vi "Chart-Draw Bounding.vi"(8 "error in (no error)":errorcluster, 11 "XY Graph Ref In":refnum<vi>) -> (0 "error out":errorcluster, 3 "XY Graph Ref Out":refnum<vi>)   [LabVIEW 2020]
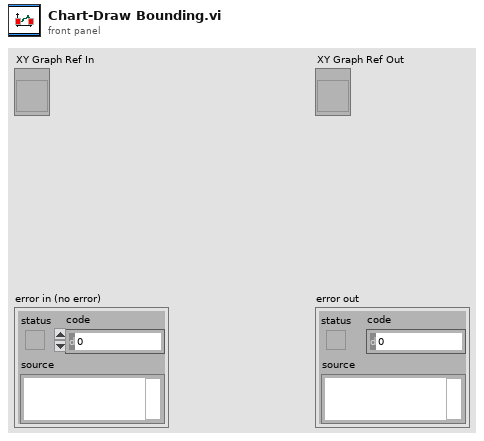
[diagram p1: front panel]
types:
  T1 = cluster{"left":i16, "top":i16, "right":i16, "bottom":i16}
  T2 = cluster{"XScale.Maximum":dbl, "XScale.Maximum":dbl}
  T3 = cluster{"XScale.Minimum":dbl, "XScale.Minimum":dbl}
  T4 = cluster{"Cursor.Cursor X":dbl, "Cursor.Cursor X":dbl}
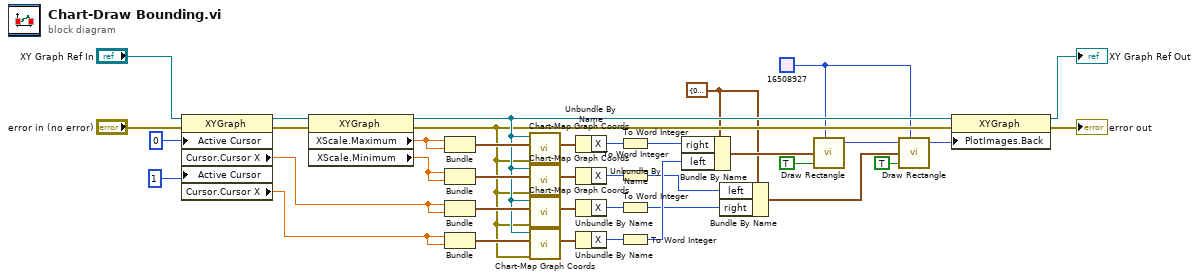
[diagram p0: block diagram]
diagram:
  w3 = u32 16508927
  w6 = T1 {"left"=0, "top"=0, "right"=0, "bottom"=500} ("rect")
  n1 = property class="XYGraph"(reference="XY Graph Ref In", error in="error in (no error)", "Active Cursor"=u32 0, "Active Cursor"=u32 1) -> (reference out=w18:refnum<vi>, error out=w19:errorcluster, "Cursor.Cursor X"=w25:dbl, "Cursor.Cursor X"=w24:dbl)
  n2 = property on="Property Node" class="XYGraph"(reference=w18, error in=w19) -> (reference out=w26:refnum<vi>, error out=w15:errorcluster, "XScale.Maximum"=w36:dbl, "XScale.Minimum"=w35:dbl)
  n3 = Bundle("XScale.Maximum"=w36, "XScale.Maximum"=w36) -> (w27:T2)  [unwired: 1 in]
  n4 = Bundle("XScale.Minimum"=w35, "XScale.Minimum"=w35) -> (w33:T3)  [unwired: 1 in]
  n5 = Bundle("Cursor.Cursor X"=w25, "Cursor.Cursor X"=w25) -> (w31:T4)  [unwired: 1 in]
  n6 = Bundle("Cursor.Cursor X"=w24, "Cursor.Cursor X"=w24) -> (w30:T4)  [unwired: 1 in]
  n7 = call "Chart-Map Graph Coords.vi"("error in (no error)"=w15, "XY"=w27, "XY Graph Ref"=w26) -> ("Coords"=w28:cluster{"X":i32, "Y":i32})  [unwired: 7 in, 1 out]
  n8 = call "Chart-Map Graph Coords.vi"("error in (no error)"=w15, "XY"=w33, "XY Graph Ref"=w26) -> ("Coords"=w34:cluster{"X":i32, "Y":i32})  [unwired: 7 in, 1 out]
  n9 = call "Chart-Map Graph Coords.vi"("error in (no error)"=w15, "XY"=w31, "XY Graph Ref"=w26) -> ("Coords"=w32:cluster{"X":i32, "Y":i32})  [unwired: 7 in, 1 out]
  n10 = call "Chart-Map Graph Coords.vi"("error in (no error)"=w15, "XY"=w30, "XY Graph Ref"=w26) -> ("Coords"=w29:cluster{"X":i32, "Y":i32})  [unwired: 7 in, 1 out]
  n11 = Unbundle By Name(w28) -> ("X"=w14:i32)
  n12 = Unbundle By Name(w34) -> ("X"=w10:i32)
  n13 = Unbundle By Name(w32) -> ("X"=w8:i32)
  n14 = Unbundle By Name(w29) -> ("X"=w12:i32)
  n15 = To Word Integer(number=w14) -> (16bit integer=w13:i16)
  n16 = To Word Integer(number=w10) -> (16bit integer=w9:i16)
  n17 = To Word Integer(number=w8) -> (16bit integer=w7:i16)
  n18 = To Word Integer(number=w12) -> (16bit integer=w11:i16)
  n19 = Bundle By Name(cluster=w6, "right"=w13, "left"=w11) -> (w23:T1)
  n20 = Bundle By Name(cluster=w6, "left"=w9, "right"=w7) -> (w5:T1)
  n21 = call <vilib>:"Draw Rectangle.vi"("rect"=w23, "fill?(F)"=TRUE, "color(black)"=w3) -> ("new picture"=w22:picture)  [unwired: 6 in]
  n22 = call <vilib>:"Draw Rectangle.vi"("picture"=w22, "rect"=w5, "fill?(F)"=TRUE, "color(black)"=w3) -> ("new picture"=w21:picture)  [unwired: 5 in]
  n23 = property on="Property Node" class="XYGraph"(reference=w26, error in=w15, "PlotImages.Back"=w21) -> (reference out=→"XY Graph Ref Out":refnum<vi>, error out=→"error out":errorcluster)
